vi "onStop.vi"(8 "error in (no error)":errorcluster, 11 "SMO":refnum<class "SMO.lvclass">) -> (0 "error out":errorcluster, 3 "SMO out":refnum<class "SMO.lvclass">)   [LabVIEW 2019, in "SMO.lvclass"]
doc: "JKI State Machine Objects (SMO) 1.3.0.56\nJKI - JKI\nCopyright (c) 2017, JKI"
uses:
  SMO.lvclass
  Typedefs/SMO Dependency--Cluster.ctl
  Typedefs/SMO Dependency Event--Enum.ctl
  Typedefs/SMO Dependency Event--Cluster.ctl
  Support/Attribute.Owner/Attribute.Owner.lvclass
panel:
  # "For instructions on how to use the JKI State Machine Objects, examples and video tutorials, visit:\nhttp://jki.net/state-machine-objects/\n\nJKI State Machine Objects™\nhttp://jki.net/state-machine-objects/\nCopyright (C) 2005-2015, JKI <info@jki.net>\nALL RIGHTS RESERVED"
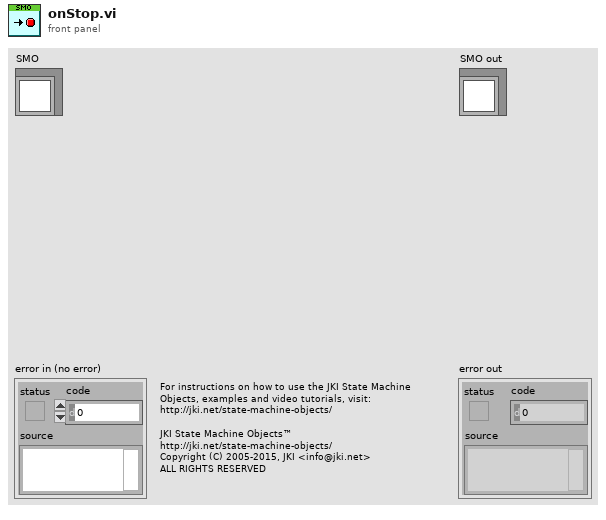
[diagram p1: front panel]
types:
  T1 = typedef "SMO.lvclass/SMO Dependency Event--Cluster.ctl" = cluster{"Name":string, "GUID":string, "Event":T2}
  T2 = typedef "SMO.lvclass/SMO Dependency Event--Enum.ctl" = enum16{"Added", "Removed", "Started", "Stopped"}
  T3 = typedef "SMO.lvclass/SMO Dependency--Cluster.ctl" = cluster{"Dependency":refnum<class "SMO.lvclass">, "Level":string}
  T4 = typedef "SMO.lvclass/PrivateData--Ref.ctl" = refnum<data-value>
  T5 = typedef "SMO.lvclass/PrivateData--Cluster.ctl" = cluster{"Parent Call":T6, "Registered Processes":T7[], "Sync Notifier":refnum<notifier>, "Process Error Notifier":refnum<notifier>, "Protected Events":T8, "Public Events":T9, "SMO State":T10, "[Dependencies]":T3[], "[Attributes]":refnum<class "Attribute.lvclass">[], "Launcher Close":refnum<notifier>, "Caller Watchdog":refnum<queue>, "Accessibility":T11, "NbStaticDependencies":u32}
  T6 = typedef "SMO.lvclass/Parent Call--Enum.ctl" = enum16{"Allows parent to run", "Does not request parent to run"}
  T7 = typedef "SMO.lvclass/RegisteredProcessData--Cluster.ctl" = cluster{"Name":string, "Static VI Ref":refnum<vi>, "Running":bool, "NotifierRef":u32}
  T8 = typedef "SMO.lvclass/Protected Events.ctl" = cluster{"StopProcesses":refnum<user-event>, "AbortProcesses":refnum<user-event>, "Config Changed":refnum<user-event>, "Dependency":refnum<user-event>}
  T9 = typedef "SMO.lvclass/Public Events.ctl" = cluster{"Error":refnum<user-event>, "State":refnum<user-event>, "Reserve State":refnum<user-event>}
  T10 = typedef "SMO.lvclass/SMOState --Enum.ctl" = enum16{"unknown", "Created", "Started", "Stopped"}
  T11 = typedef "SMO.lvclass/Accessibility--Cluster.ctl" = cluster{"Lock Key":string, "Reserve State":T12}
  T12 = typedef "SMO.lvclass/Reserve State--Enum.ctl" = enum16{"Unreserved", "Reserved", "Self-locked"}
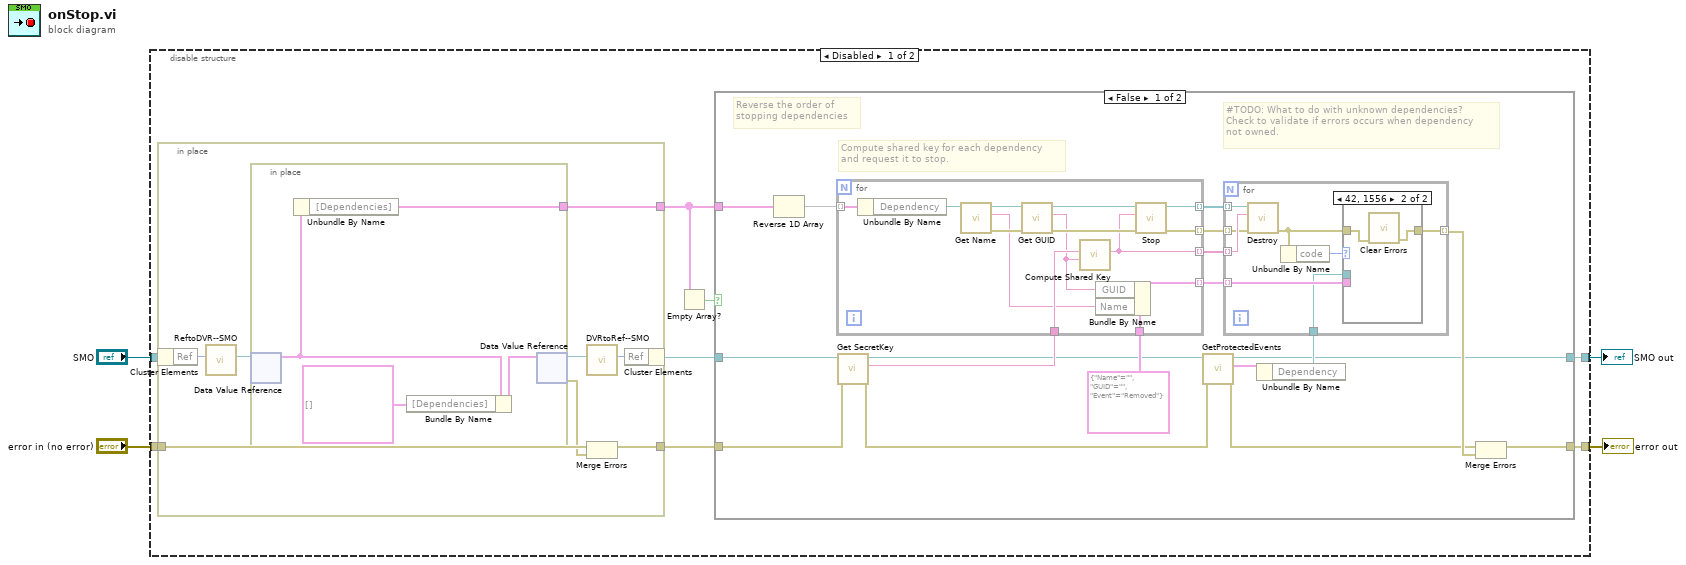
[diagram p0: block diagram]
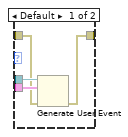
[diagram p2: hidden frame]
diagram:
  n1 = disable-structure shown="Disabled" {
    disable-tunnel: "SMO" -> [w8 w74]
    disable-tunnel: "error in (no error)" -> [w7 w73]
    disable-tunnel: [w6 w74] -> w2
    disable-tunnel: [w5 w73] -> w1
    frame Disabled {
      n2 = in-place {
        in-place-border: w7 -> [w64]
        in-place-border: [w62] -> w11
        in-place-border: [w61] -> w9
        n3 = in-place-cluster #1(w8) -> ("Ref"=w68:u32)
        n4 = call "ReftoDVR--SMO.vi"("Ref"=w68) -> ("Ref"=w67:T4)  [unwired: 10 in]
        n5 = in-place {
          in-place-border: [w72] -> w61
          n6 = in-place-dvr #2(w67) -> (w71:T5)  [unwired: 1 out]
          n7 = Unbundle By Name(w71) -> ("[Dependencies]"=w72:T3[])
          n8 = Bundle By Name(cluster=w71, "[Dependencies]"=T3[] []) -> (w70:T5)
          n9 = in-place-dvr #2(w70) -> (w66:T4, w63:errorcluster)
        }
        n10 = call "DVRtoRef--SMO.vi"("Ref"=w66) -> ("Ref"=w65:u32)  [unwired: 10 in]
        n11 = Merge Errors(w64, w63) -> (w62:errorcluster)
        n12 = in-place-cluster #1("Ref"=w65) -> (w12:refnum<class "SMO.lvclass">)
      }
      n13 = Empty Array?(array=w9) -> (empty?=w10:bool)
      n14 = case shown="False" w10 {
        tunnel: [w30 w59] -> w5
        tunnel: w9 -> [w29 _]
        tunnel: w12 -> [w28 w60]
        tunnel: w11 -> [w27 w59]
        tunnel: [w13 w60] -> w6
        frame False {
          # "#TODO: What to do with unknown dependencies?\nCheck to validate if errors occurs when dependency\nnot owned."
          # "Reverse the order of\nstopping dependencies"
          # "Compute shared key for each dependency\nand request it to stop."
          n15 = Reverse 1D Array(array=w29) -> (reversed array=w25:T3[])
          n16 = call "Get SecretKey.vi"("error in (no error)"=w27, "SMO"=w28) -> ("error out"=w17:errorcluster, "SecretKey"=w26:string, "SMO out"=w18:refnum<class "SMO.lvclass">)  [unwired: 7 in]
          n17 = for {
            tunnel: w25 -> [w55] mode=indexing
            tunnel: w26 -> [w57]
            tunnel: [w54] -> w24 mode=indexing
            tunnel: [w53] -> w23 mode=indexing
            tunnel: [w52] -> w22 mode=indexing
            tunnel: T1 {"Name"="", "GUID"="", "Event"=enum."Removed"} ("Dependency Event") -> [w46]
            tunnel: [w45] -> w19 mode=indexing
            n18 = Unbundle By Name(w55) -> ("Dependency"=w51:refnum<class "SMO.lvclass">)
            n19 = call "Get Name.vi"("SMO"=w51) -> ("error out"=w49:errorcluster, "Name"=w47:string, "SMO out"=w50:refnum<class "SMO.lvclass">)  [unwired: 8 in]
            n20 = call "Get GUID.vi"("error in (no error)"=w49, "SMO"=w50) -> ("error out"=w56:errorcluster, "GUID"=w48:string, "SMO out"=w58:refnum<class "SMO.lvclass">)  [unwired: 7 in]
            n21 = call "Compute Shared Key.vi"("GUID"=w48, "SecretKey"=w57) -> ("Shared Key"=w53:string)  [unwired: 9 in]
            n22 = Bundle By Name(cluster=w46, "GUID"=w48, "Name"=w47) -> (w45:T1)
            n23 = call "Stop.vi"("error in (no error)"=w56, "Shared Key"=w53, "SMO"=w58) -> ("error out"=w52:errorcluster, "SMO out"=w54:refnum<class "SMO.lvclass">)  [unwired: 7 in]
          }
          n24 = call "GetProtectedEvents.vi"("error in (no error)"=w17, "SMO"=w18) -> ("error out"=w16:errorcluster, "SMO Protected Events"=w15:T8, "SMO out"=w13:refnum<class "SMO.lvclass">)  [unwired: 7 in]
          n25 = Unbundle By Name(w15) -> ("Dependency"=w14:refnum<user-event>)
          n26 = for {
            tunnel: w24 -> [w38] mode=indexing
            tunnel: w23 -> [w37] mode=indexing
            tunnel: [w33] -> w21 mode=indexing
            tunnel: w22 -> [w36] mode=indexing
            tunnel: w19 -> [w32] mode=indexing
            tunnel: w14 -> [w31]
            n27 = call "Destroy.vi"("error in (no error)"=w36, "Shared Key"=w37, "SMO"=w38) -> ("error out"=w34:errorcluster)  [unwired: 8 in]
            n28 = Unbundle By Name(w34) -> ("code"=w35:i32)
            n29 = case shown="42, 1556" w35 {
              tunnel: w34 -> [w40 w44]
              tunnel: [w39 w43] -> w33
              tunnel: w32 -> [w41 _]
              tunnel: w31 -> [w42 _]
              frame Default {
                n30 = Generate User Event(user event=w42, event data cluster=w41, error in=w40) -> (error out=w39:errorcluster)  [unwired: 1 in, 1 out]
              }
              frame 42, 1556 {
                n31 = call <vilib>:"Clear Errors.vi"("error in (no error)"=w44) -> ("error out"=w43:errorcluster)  [unwired: 5 in, 1 out]
              }
            }
          }
          n32 = Merge Errors(w16, w21) -> (w30:errorcluster)
        }
        frame True {
        }
      }
    }
    frame Enabled {
    }
  }
  "error out" <- w1
  "SMO out" <- w2
